vi "ZMQ.Connect.vi"(8 "error in (no error)":errorcluster, 11 "RemoteControl.ZMQ in":refnum<class "RemoteControl.ZMQ.lvclass">) -> (0 "error out":errorcluster, 3 "RemoteControl.ZMQ out":refnum<class "RemoteControl.ZMQ.lvclass">)   [LabVIEW 2019, in "RemoteControl.ZMQ.lvclass"]
uses:
  RemoteControl.ZMQ.lvclass
  RemoteControl.ZMQ.lvclass/RemoteControl.ZMQ.ctl
  <vilib>/addons/zeromq/zeromq.lvlib
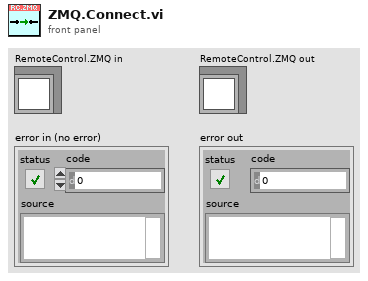
[diagram p1: front panel]
types:
  T1 = typedef "zeromq.lvlib/socket_type.ctl" = enum8{"ZMQ_PAIR", "ZMQ_PUB", "ZMQ_SUB", "ZMQ_REQ", "ZMQ_REP", "ZMQ_DEALER", "ZMQ_ROUTER", "ZMQ_PULL", "ZMQ_PUSH", "ZMQ_XPUB", "ZMQ_XSUB", "ZMQ_STREAM", "ZMQ_SERVER", "ZMQ_CLIENT", "ZMQ_RADIO", "ZMQ_DISH", "ZMQ_GATHER", "ZMQ_SCATTER", "ZMQ_DGRAM"}
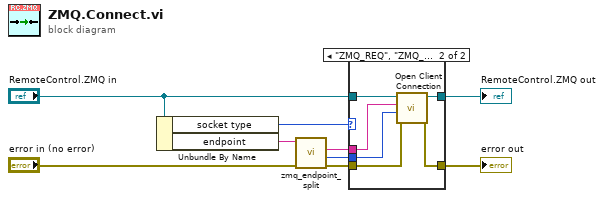
[diagram p0: block diagram]
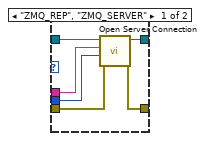
[diagram p2: hidden frame]
diagram:
  n1 = Unbundle By Name("RemoteControl.ZMQ in") -> ("socket type"=w1:T1, "endpoint"=w4:string)
  n2 = call <vilib>:"zmq_endpoint_split.vi"("error in"="error in (no error)", "endpoint"=w4) -> ("error out"=w7:errorcluster, "port"=w2:u16, "address"=w3:string)  [unwired: 2 in, 1 out]
  n3 = case shown="\"ZMQ_REQ\", \"ZMQ_CLIENT\", Default" w1 {
    tunnel: "RemoteControl.ZMQ in" -> [w15 w21]
    tunnel: [w14 w20] -> w5
    tunnel: w2 -> [w12 w19]
    tunnel: w3 -> [w13 w18]
    tunnel: w7 -> [w11 w17]
    tunnel: [w10 w16] -> w9
    frame "ZMQ_REP", "ZMQ_SERVER" {
      n4 = call-dynamic "Open Server Connection.vi"("error in (no error)"=w11, "Port"=w12, "address"=w13, "RemoteControl.ZMQ in"=w15) -> ("error out"=w10:errorcluster, "RemoteControl.ZMQ out"=w14:refnum<class "RemoteControl.ZMQ.lvclass">)  [unwired: 6 in]
    }
    frame "ZMQ_REQ", "ZMQ_CLIENT", Default {
      n5 = call-dynamic "Open Client Connection.vi"("error in (no error)"=w17, "Port"=w19, "address"=w18, "RemoteControl.ZMQ in"=w21) -> ("error out"=w16:errorcluster, "RemoteControl.ZMQ out"=w20:refnum<class "RemoteControl.ZMQ.lvclass">)  [unwired: 6 in]
    }
  }
  "error out" <- w9
  "RemoteControl.ZMQ out" <- w5
